vi "ConfigXMLCore.vi"(9 "ConnectionData":T1, 10 "controlsToSave":refnum<vi>[](array[refnum]), 11 "ConfigXMLControl":T2) -> ()   [LabVIEW 2015]
uses:
  ConfigXMLControl.ctl
  General/RemoteFiles/connectionData.ctl
panel:
  out "robotIP":string
  # "Core controller VI for the XML config plugin.\nhandles all saving, loading, file transfer, etc."
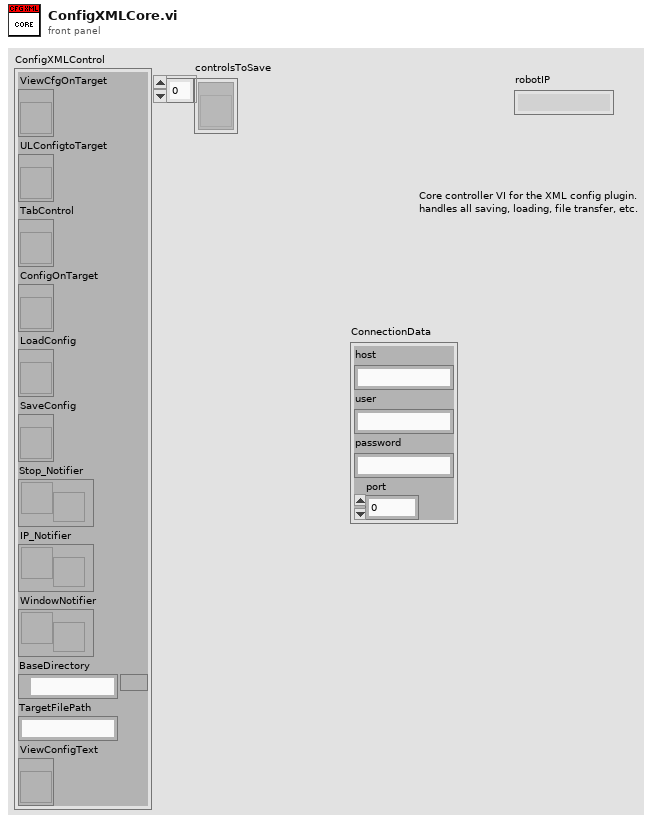
[diagram p1: front panel]
types:
  T1 = typedef "connectionData.ctl" = cluster{"host":string, "user":string, "password":string, "port":u16}
  T2 = typedef "ConfigXMLControl.ctl" = cluster{"ViewCfgOnTarget":refnum<vi>, "ULConfigtoTarget":refnum<vi>, "TabControl":refnum<vi>, "ConfigOnTarget":refnum<vi>, "LoadConfig":refnum<vi>, "SaveConfig":refnum<vi>, "Stop_Notifier":refnum<notifier>, "IP_Notifier":refnum<notifier>, "WindowNotifier":refnum<notifier>, "BaseDirectory":path, "TargetFilePath":string, "ViewConfigText":refnum<vi>}
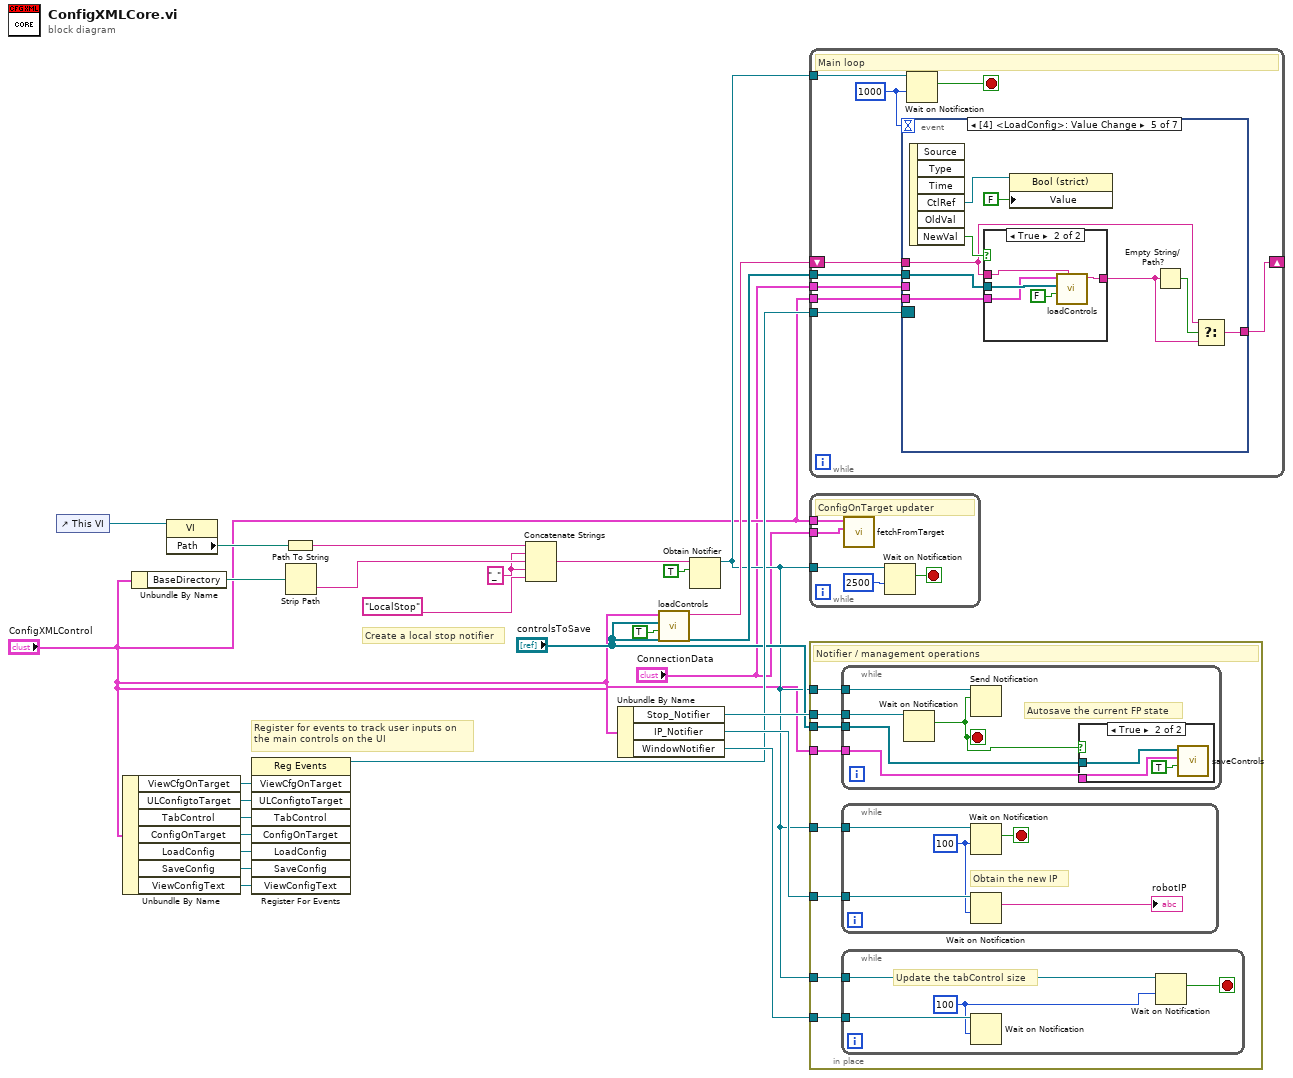
[diagram p0: block diagram]
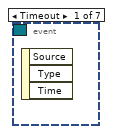
[diagram p2: hidden frame]
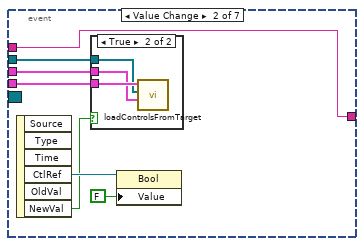
[diagram p3: hidden frame]
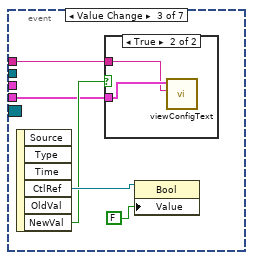
[diagram p5: hidden frame]
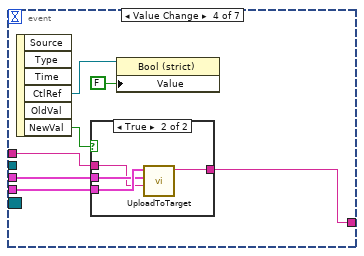
[diagram p7: hidden frame]
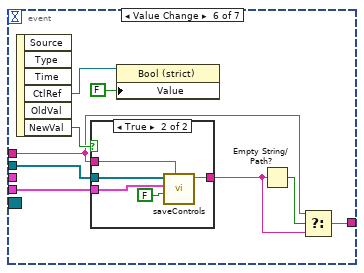
[diagram p10: hidden frame]
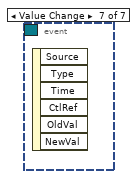
[diagram p12: hidden frame]
diagram:
  w11 = "_" ("string")
  # "Create a local stop notifier"
  # "Register for events to track user inputs on\nthe main controls on the UI"
  n1 = control-ref of="This VI"() -> (w16:refnum<vi>)
  n2 = Unbundle By Name("ConfigXMLControl") -> ("ViewCfgOnTarget"=w23:refnum<vi>, "ULConfigtoTarget"=w22:refnum<vi>, "TabControl"=w21:refnum<vi>, "ConfigOnTarget"=w20:refnum<vi>, "LoadConfig"=w19:refnum<vi>, "SaveConfig"=w18:refnum<vi>, "ViewConfigText"=w1:refnum<vi>)
  n3 = Unbundle By Name("ConfigXMLControl") -> ("BaseDirectory"=w14:path)
  n4 = property class="VI"(reference=w16) -> ("Path"=w15:path)  [unwired: 1 in, 2 out]
  n5 = register-events(w23, w22, w21, w20, w19, w18, w1) -> (reference out=w17:refnum<event-registration>)  [unwired: 2 in, 1 out]
  n6 = Path To String(path=w15) -> (string=w13:string)
  n7 = Strip Path(path=w14) -> (name=w12:string)  [unwired: 1 out]
  n8 = Concatenate Strings(w13, w11, w12, w11, "LocalStop" ("string")) -> (w9:string)
  n9 = Unbundle By Name("ConfigXMLControl") -> ("Stop_Notifier"=w26:refnum<notifier>, "IP_Notifier"=w25:refnum<notifier>, "WindowNotifier"=w24:refnum<notifier>)
  n10 = call "loadControls.vi"("Autoload?"=TRUE, "ControlsToLoad"="controlsToSave", "ConfigXMLControls"="ConfigXMLControl") -> ("nameUsed"=w6:string)  [unwired: 7 in, 1 out]
  n11 = Obtain Notifier(name (unnamed)=w9, notification data type=TRUE) -> (notifier out=w4:refnum<notifier>)  [unwired: 2 in, 2 out]
  n12 = while {
    tunnel: w17 -> [w35]
    tunnel: "ConfigXMLControl" -> [w34]
    tunnel: "controlsToSave" -> [w33]
    tunnel: w4 -> [w31]
    shift-right: [w29] -> _
    shift-left: w6 -> [w30]
    tunnel: "ConnectionData" -> [w28]
    stop <- w32 stop-if-true
    w27 = 1000
    # "Main loop"
    n13 = event shown="[4] <LoadConfig>: Value Change" {
      selector: w35 -> [_ _ _ _ _ _ _]
      dyn-events: _ -> [_ _ _ _ _ _ _]
      timeout: w27 -> [_ _ _ _ _ _ _]
      tunnel: w34 -> [_ w39 w47 w56 w71 w84 _]
      tunnel: w33 -> [_ w37 _ _ w72 w83 _]
      tunnel: w30 -> [_ w36 w46 w54 w66 w79 _]
      tunnel: [_ w36 _ w53 w65 w80 _] -> w29
      tunnel: w28 -> [_ w38 _ w55 _ _ _]
      event Timeout {
        n14 = event-data() -> ()  [unwired: 1 in, 3 out]
      }
      event Value Change {
        n15 = event-data() -> ("CtlRef"=w41:refnum<vi>, "NewVal"=w40:bool)  [unwired: 1 in, 4 out]
        n16 = case shown="True" w40 {
          tunnel: w39 -> [_ w45]
          tunnel: w38 -> [_ w44]
          tunnel: w37 -> [_ w43]
          frame False {
          }
          frame True {
            n17 = call "loadControlsFromTarget.vi"("ConnectionData"=w44, "ControlsToLoad"=w43, "ConfigXMLControls"=w45) -> ()  [unwired: 8 in, 1 out]
          }
        }
        n18 = property class="Bool"(reference=w41, "Value"=FALSE) -> ()  [unwired: 1 in, 2 out]
      }
      event Value Change {
        n19 = event-data() -> ("CtlRef"=w50:refnum<vi>, "NewVal"=w48:bool)  [unwired: 1 in, 4 out]
        n20 = case shown="True" w48 {
          tunnel: w47 -> [_ w52]
          tunnel: w46 -> [_ w51]
          frame False {
          }
          frame True {
            n21 = call "viewConfigText.vi"("prevName"=w51, "ConfigXMLControls"=w52) -> ()  [unwired: 9 in, 1 out]
          }
        }
        n22 = property class="Bool"(reference=w50, "Value"=FALSE) -> ()  [unwired: 1 in, 2 out]
      }
      event Value Change {
        n23 = event-data() -> ("CtlRef"=w59:refnum<vi>, "NewVal"=w57:bool)  [unwired: 1 in, 4 out]
        n24 = case shown="True" w57 {
          tunnel: w56 -> [_ w64]
          tunnel: w55 -> [_ w63]
          tunnel: w54 -> [w60 w62]
          tunnel: [w60 w61] -> w53
          frame False {
          }
          frame True {
            n25 = call "UploadToTarget.vi"("previousName"=w62, "ConnectionData"=w63, "ConfigXMLControls"=w64) -> ("newName"=w61:string)  [unwired: 7 in, 1 out]
          }
        }
        n26 = property class="Bool (strict)"(reference=w59, "Value"=FALSE) -> ()  [unwired: 1 in, 2 out]
      }
      event Value Change {
        n27 = event-data() -> ("CtlRef"=w70:refnum<vi>, "NewVal"=w69:bool)  [unwired: 1 in, 4 out]
        n28 = case shown="True" w69 {
          tunnel: w71 -> [_ w76]
          tunnel: w72 -> [_ w78]
          tunnel: [_ w75] -> w67
          tunnel: w66 -> [_ w74]
          frame False {
          }
          frame True {
            n29 = call "loadControls.vi"("prevName"=w74, "Autoload?"=FALSE ("isAutoSave"), "ControlsToLoad"=w78, "ConfigXMLControls"=w76) -> ("nameUsed"=w75:string)  [unwired: 6 in, 1 out]
          }
        }
        n30 = property class="Bool (strict)"(reference=w70, "Value"=FALSE) -> ()  [unwired: 1 in, 2 out]
        n31 = Empty String/Path?(string/path=w67) -> (empty?=w68:bool)
        n32 = Select(t=w66, s=w68, f=w67) -> (s? t:f=w65:string)
      }
      event Value Change {
        n33 = event-data() -> ("CtlRef"=w87:refnum<vi>, "NewVal"=w85:bool)  [unwired: 1 in, 4 out]
        n34 = case shown="True" w85 {
          tunnel: w84 -> [_ w92]
          tunnel: w83 -> [_ w91]
          tunnel: [_ w89] -> w81
          tunnel: w79 -> [_ w88]
          frame False {
          }
          frame True {
            n35 = call "saveControls.vi"("prevName"=w88, "isAutoSave"=FALSE, "ConfigXMLControls"=w92, "ControlsToSave"=w91) -> ("nameUsed"=w89:string)  [unwired: 6 in, 1 out]
          }
        }
        n36 = property class="Bool (strict)"(reference=w87, "Value"=FALSE) -> ()  [unwired: 1 in, 2 out]
        n37 = Empty String/Path?(string/path=w81) -> (empty?=w82:bool)
        n38 = Select(t=w79, s=w82, f=w81) -> (s? t:f=w80:string)
      }
      event Value Change {
        n39 = event-data() -> ()  [unwired: 1 in, 6 out]
      }
    }
    n40 = Wait on Notification(notifier=w31, timeout in ms (-1)=w27) -> (notification=w32:bool)  [unwired: 2 in, 3 out]
  }
  n41 = while {
    tunnel: w4 -> [w95]
    tunnel: "ConfigXMLControl" -> [w94]
    tunnel: "ConnectionData" -> [w93]
    stop <- w96 stop-if-true
    # "ConfigOnTarget updater"
    n42 = call "fetchFromTarget.vi"("ConnectionData"=w93, "ConfigXMLControls"=w94) -> ()  [unwired: 5 in, 5 out]
    n43 = Wait on Notification(notifier=w95, timeout in ms (-1)=2500) -> (notification=w96:bool)  [unwired: 2 in, 3 out]
  }
  n44 = in-place {
    in-place-border: w26 -> [w105]
    in-place-border: w25 -> [w104]
    in-place-border: w24 -> [w103]
    in-place-border: "ConfigXMLControl" -> [w102]
    in-place-border: "controlsToSave" -> [w101]
    in-place-border: w4 -> [w100]
    in-place-border: w4 -> [w99]
    in-place-border: w4 -> [w98]
    # "Notifier / management operations"
    n45 = while {
      tunnel: w105 -> [w119]
      tunnel: w102 -> [w118]
      tunnel: w101 -> [w117]
      tunnel: w100 -> [w116]
      stop <- w115 stop-if-true
      # "Autosave the current FP state"
      n46 = Wait on Notification(notifier=w119) -> (notification=w115:bool)  [unwired: 3 in, 3 out]
      n47 = Send Notification(notification=w115, notifier=w116) -> ()  [unwired: 1 in, 2 out]
      n48 = case shown="True" w115 {
        tunnel: w118 -> [_ w122]
        tunnel: w117 -> [_ w121]
        frame False {
        }
        frame True {
          n49 = call "saveControls.vi"("isAutoSave"=TRUE, "ConfigXMLControls"=w122, "ControlsToSave"=w121) -> ()  [unwired: 7 in, 2 out]
        }
      }
    }
    n50 = while {
      tunnel: w104 -> [w114]
      tunnel: w99 -> [w112]
      stop <- w111 stop-if-true
      w110 = 100 ("timeout in ms (-1)")
      # "Obtain the new IP"
      n51 = Wait on Notification(notifier=w112, timeout in ms (-1)=w110) -> (notification=w111:bool)  [unwired: 2 in, 3 out]
      n52 = Wait on Notification(notifier=w114, timeout in ms (-1)=w110) -> (notification=→"robotIP":string)  [unwired: 2 in, 3 out]
    }
    n53 = while {
      tunnel: w103 -> [w109]
      tunnel: w98 -> [w107]
      stop <- w106 stop-if-true
      w108 = 100 ("timeout in ms (-1)")
      # "Update the tabControl size"
      n54 = Wait on Notification(notifier=w109, timeout in ms (-1)=w108) -> ()  [unwired: 2 in, 4 out]
      n55 = Wait on Notification(notifier=w107, timeout in ms (-1)=w108) -> (notification=w106:bool)  [unwired: 2 in, 3 out]
    }
  }
